vi "менеджер.vi"(8 "task":T1(ring), 10 "дані":variant, 11 "queue":refnum<queue>) -> (0 "дані вихід":variant, 3 "queue out":refnum<queue>)   [LabVIEW 2013]
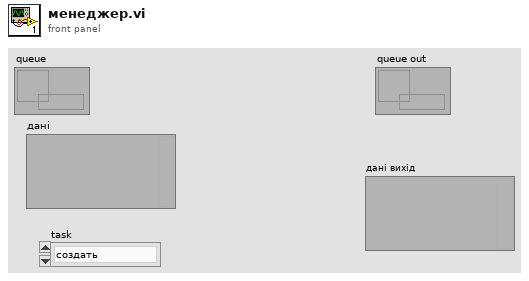
[diagram p1: front panel]
types:
  T1 = enum16{"создать", "добавить в начало", "добавить в конец", "считать", "очистить", "удалить", "пустий", ""}
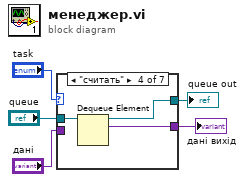
[diagram p0: block diagram]
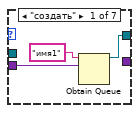
[diagram p2: hidden frame]
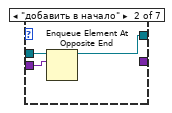
[diagram p3: hidden frame]
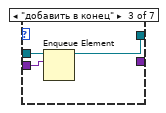
[diagram p4: hidden frame]
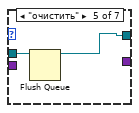
[diagram p5: hidden frame]
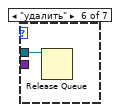
[diagram p6: hidden frame]
diagram:
  n1 = case shown="\"считать\"" "task" {
    tunnel: "queue" -> [_ w11 w14 w17 w19 w20 w21]
    tunnel: "дані" -> [w8 w10 w13 _ _ _ _]
    tunnel: [_ _ _ w16 _ _ _] -> w2
    tunnel: [w6 w9 w12 w15 w18 _ w21] -> w1
    frame "создать" {
      n2 = Obtain Queue(name (unnamed)="имя1", element data type=w8) -> (queue out=w6:refnum<queue>)  [unwired: 3 in, 2 out]
    }
    frame "добавить в начало" {
      n3 = Enqueue Element At Opposite End(queue=w11, element=w10) -> (queue out=w9:refnum<queue>)  [unwired: 2 in, 2 out]
    }
    frame "добавить в конец" {
      n4 = Enqueue Element(queue=w14, element=w13) -> (queue out=w12:refnum<queue>)  [unwired: 2 in, 2 out]
    }
    frame "считать" {
      n5 = Dequeue Element(queue=w17) -> (queue out=w15:refnum<queue>, element=w16:variant)  [unwired: 2 in, 2 out]
    }
    frame "очистить" {
      n6 = Flush Queue(queue=w19) -> (queue out=w18:refnum<queue>)  [unwired: 1 in, 2 out]
    }
    frame "удалить" {
      n7 = Release Queue(queue=w20) -> ()  [unwired: 2 in, 3 out]
    }
    frame "пустий", Default {
    }
  }
  "дані вихід" <- w2
  "queue out" <- w1
